vi "Przenies opisy FVG.vi"(7 "Akcja (Get)":T1, 8 "error in (no error)":errorcluster, 10 "DI opisy in":string[](array[string]), 11 "AI opisy in":string[](array[string])) -> (0 "error out":errorcluster, 2 "DI opisy out":string[](array[string]), 3 "AI opisy out":string[](array[string]))   [LabVIEW 2013]
doc: "Zmienna funkcjonalna przenosząca nazwy\nkanałów AI oraz DI\nz pętli GUI do pętli ACQ"
uses:
  Kontrolki/FVGs/FVG GUI akcje.ctl
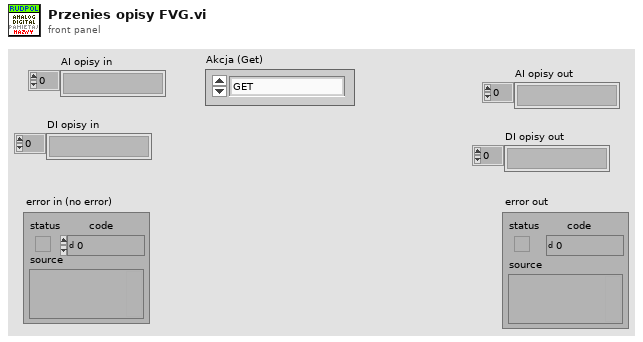
[diagram p1: front panel]
types:
  T1 = typedef "FVG GUI akcje.ctl" = enum16{"GET", "SET AI Aktywny", "SET DI Aktywny"}
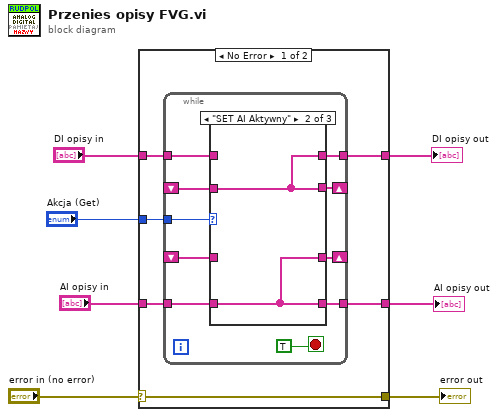
[diagram p0: block diagram]
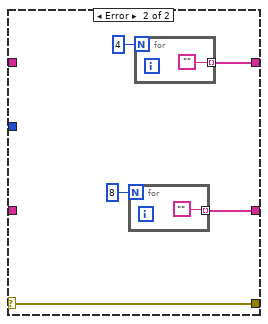
[diagram p4: hidden frame]
diagram:
  n1 = case shown="No Error" "error in (no error)" {
    selector: "error in (no error)" -> [w13 w34]
    tunnel: [w13 w34] -> w6
    tunnel: "AI opisy in" -> [w12 _]
    tunnel: [w11 w32] -> w3
    tunnel: "DI opisy in" -> [w10 _]
    tunnel: "Akcja (Get)" -> [w9 _]
    tunnel: [w8 w30] -> w1
    frame No Error {
      n2 = while {
        tunnel: w9 -> [w22]
        tunnel: w12 -> [w21]
        shift-right: [w20] -> _
        shift-left: _ -> [w19]
        tunnel: [w18] -> w11
        tunnel: w10 -> [w17]
        shift-right: [w16] -> _
        shift-left: _ -> [w14]
        tunnel: [w15] -> w8
        stop <- TRUE stop-if-true
        n3 = case shown="\"SET AI Aktywny\"" w22 {
          tunnel: w21 -> [_ w27 _]
          tunnel: [w25 w27 w29] -> w20
          tunnel: w19 -> [w25 _ w29]
          tunnel: [w25 w27 w29] -> w18
          tunnel: w17 -> [_ _ w28]
          tunnel: [w24 w26 w28] -> w16
          tunnel: [w24 w26 w28] -> w15
          tunnel: w14 -> [w24 w26 _]
          frame "GET", Default {
          }
          frame "SET AI Aktywny" {
          }
          frame "SET DI Aktywny" {
          }
        }
      }
    }
    frame Error {
      n4 = for {
        N: 8 -> [_]
        tunnel: [""] -> w32 mode=indexing
      }
      n5 = for {
        N: 4 -> [_]
        tunnel: [""] -> w30 mode=indexing
      }
    }
  }
  "error out" <- w6
  "AI opisy out" <- w3
  "DI opisy out" <- w1
